vi "FTW-Endpoint-Bind-Async.vi"(0 "FTW Endpoint":refnum<class "FTW-Actor-Endpoint.lvclass">, 5 "Endpoint Address":string, 11 "error in":errorcluster) -> (4 "FTW Endpoint out":refnum<class "FTW-Actor-Endpoint.lvclass">, 6 "Actual Endpoint Address":string, 8 "Incoming Message":refnum<event-registration>, 15 "error out":errorcluster)   [LabVIEW 2013, in "FTW-Actor-Endpoint.lvclass"]
uses:
  FTW-Actor-Endpoint.lvclass
  request/FTW-Request.lvclass
panel:
  # "Inputs"
  # "Outputs"
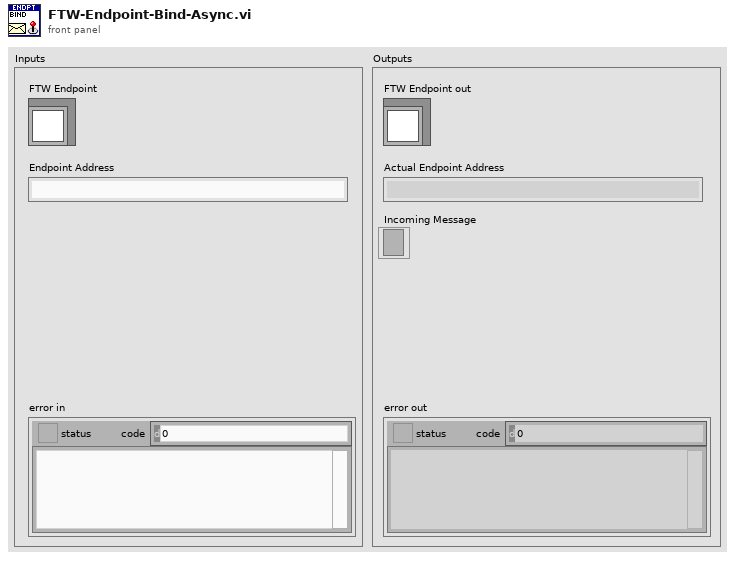
[diagram p1: front panel]
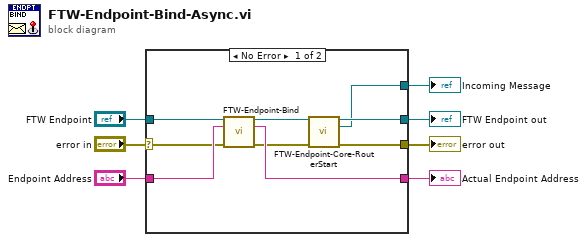
[diagram p0: block diagram]
diagram:
  n1 = case shown="No Error" "error in" {
    selector: "error in" -> [w13 w18]
    tunnel: [w10 w18] -> w7
    tunnel: [w9 w17] -> w5
    tunnel: "FTW Endpoint" -> [w16 w17]
    tunnel: "Endpoint Address" -> [w15 _]
    tunnel: [w14 _] -> w2
    tunnel: [w8 _] -> w1
    frame No Error {
      n2 = call-dynamic "FTW-Endpoint-Bind.vi"("FTW Endpoint"=w16, "Remote Endpoint Address"=w15, "error in"=w13) -> ("FTW Endpoint out"=w12:refnum<class "FTW-Actor-Endpoint.lvclass">, "Actual Endpoint Address"=w14:string, "error out"=w11:errorcluster)  [unwired: 10 in]
      n3 = call "FTW-Endpoint-Core-RouterStart.vi"("FTW Endpoint"=w12, "error in"=w11) -> ("FTW Endpoint out"=w9:refnum<class "FTW-Actor-Endpoint.lvclass">, "Incoming Message"=w8:refnum<event-registration>, "error out"=w10:errorcluster)  [unwired: 11 in]
    }
    frame Error {
    }
  }
  "error out" <- w7
  "FTW Endpoint out" <- w5
  "Actual Endpoint Address" <- w2
  "Incoming Message" <- w1
